vi "Main - Init Close Variables RT.vi"(6 "State":enum16{"Init", "Close"}(ring), 8 "Error In":errorcluster) -> (0 "Error Out":errorcluster)   [LabVIEW 2020]
uses:
  Control/State - eFGV.ctl
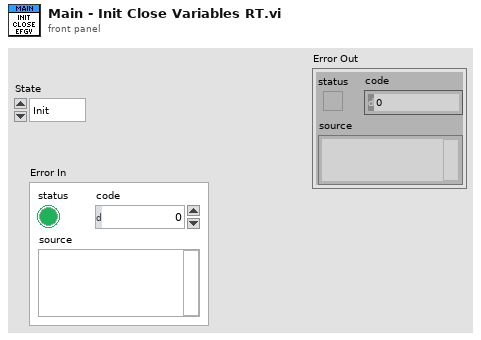
[diagram p1: front panel]
types:
  T1 = typedef "State - eFGV.ctl" = enum16{"Init", "Read", "Write", "Exit"}
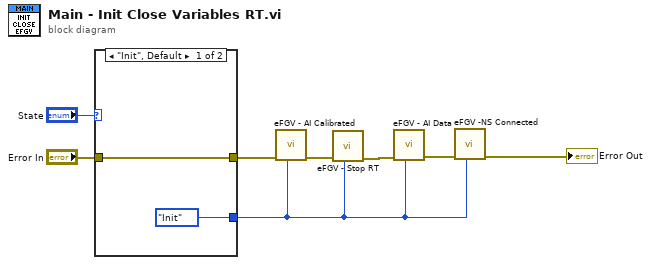
[diagram p0: block diagram]
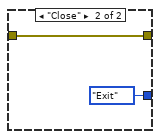
[diagram p2: hidden frame]
diagram:
  n1 = case shown="\"Init\", Default" "State" {
    tunnel: [w10 w12] -> w3
    tunnel: "Error In" -> [w10 w12]
    tunnel: [State_-_eFGV."Init" ("State - eFGV") State_-_eFGV."Exit" ("State - eFGV")] -> w2
    frame "Init", Default {
    }
    frame "Close" {
    }
  }
  n2 = call "eFGV - AI Calibrated.vi"("State"=w2, "error in (no error)"=w3) -> ("error out"=w1:errorcluster)  [unwired: 8 in, 1 out]
  n3 = call "eFGV - Stop RT.vi"("State"=w2, "Error In"=w1) -> ("Error Out"=w6:errorcluster)  [unwired: 7 in, 2 out]
  n4 = call "eFGV - AI Data.vi"("States"=w2, "Error In"=w6) -> ("Error Out"=w5:errorcluster)  [unwired: 8 in, 1 out]
  n5 = call "eFGV -NS Connected.vi"("States"=w2, "Error In"=w5) -> ("Error Out"=→"Error Out":errorcluster)  [unwired: 8 in, 1 out]
